vi "CastByteArrayAndDispatchMsg.vi"(8 "error in (no error)":errorcluster, 10 "Raw Data":i8[](array[numeric]), 11 "DIMDemoServer in":refnum<class "DIMDemoServer.lvclass">) -> (0 "error out":errorcluster, 3 "DIMDemoServer out":refnum<class "DIMDemoServer.lvclass">)   [LabVIEW 2012, in "DimActorDemo.lvlib" / "DIMDemoServer.lvclass"]
doc: "Type cast byte array to G data with respect to type descriptor and dispatch message to self."
uses:
  DIMDemoServer.lvclass
  <vilib>/ActorFramework/Actor/Actor.lvclass/Actor.ctl
  <vilib>/ActorFramework/Message Enqueuer/Message Enqueuer.lvclass/Message Enqueuer.ctl
  DIMDemoServer Messages/Update DemoService Msg/Update DemoService Msg.lvclass/Update DemoService Msg.ctl
  <vilib>/ActorFramework/Message Enqueuer/Init from Existing Queue.vi
  <vilib>/ActorFramework/Message Enqueuer/Enqueue.vi
  <vilib>/ActorFramework/Message Priority Queue/Priority Enqueue.vi
  <vilib>/ActorFramework/Message Enqueuer/Message Enqueuer.lvclass
  DIMDemoServer Messages/Update DemoService Msg/Update DemoService Msg.lvclass
  <vilib>/ActorFramework/Actor/Actor.lvclass
  SVN/LV2009/GPL/lib.lib/DimLVEvent/LVDimInterface/LVDimInterface.lvlib
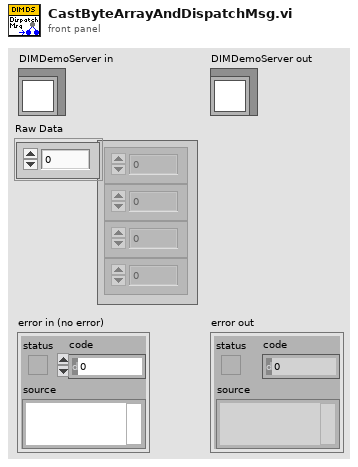
[diagram p1: front panel]
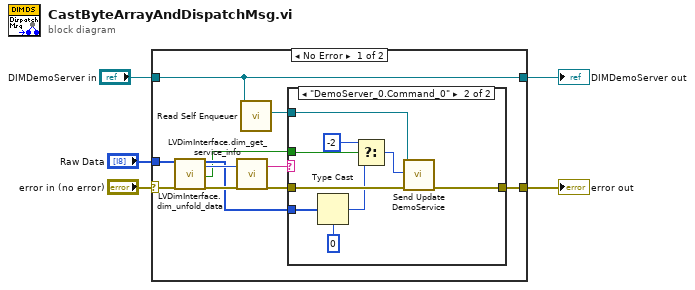
[diagram p0: block diagram]
diagram:
  n1 = case shown="No Error" "error in (no error)" {
    selector: "error in (no error)" -> [w7 w27]
    tunnel: "Raw Data" -> [w15 _]
    tunnel: "DIMDemoServer in" -> [w6 w28]
    tunnel: [w8 w27] -> w3
    tunnel: [w6 w28] -> w1
    frame No Error {
      n2 = call "LVDimInterface.dim_unfold_data.vi"("rawData"=w15, "error in (no error)"=w7) -> ("data"=w12:i8[], "callBackID"=w16:i32, "no link"=w9:bool, "error out"=w14:errorcluster)  [unwired: 14 in]
      n3 = call "LVDimInterface.dim_get_service_info.vi"("callBackID"=w16, "error in (no error)"=w14) -> ("serviceName"=w13:string, "error out"=w10:errorcluster)  [unwired: 8 in, 8 out]
      n4 = call <vilib>:"Read Self Enqueuer.vi"("Actor"=w6) -> ("Self Enqueuer"=w11:refnum<class "Message Enqueuer.lvclass">)  [unwired: 10 in]
      n5 = case shown="\"DemoServer_0.Command_0\"" w13 {
        tunnel: w12 -> [_ w25]
        tunnel: w11 -> [_ w24]
        tunnel: w10 -> [w17 w23]
        tunnel: w9 -> [_ w22]
        tunnel: [w17 w18] -> w8
        frame Default {
        }
        frame "DemoServer_0.Command_0" {
          n6 = Type Cast(type=0, x=w25) -> (*(type *) &x=w20:i32)
          n7 = Select(t=-2, s=w22, f=w20) -> (s? t:f=w19:i32)
          n8 = call "Send Update DemoService.vi"("error in (no error)"=w23, "DemoService"=w19, "Message Enqueuer"=w24) -> ("error out"=w18:errorcluster)  [unwired: 7 in, 1 out]
        }
      }
    }
    frame Error {
    }
  }
  "error out" <- w3
  "DIMDemoServer out" <- w1
